vi "Allan variance.vi"(9 "iTime":sgl[](array[numeric])=[1.0, 2.0, 5.0, 10.0, 20.0, 25.0, 50.0, 100.0, 200.0, 250.0, 500.0, 1000.0], 10 "mTime":sgl=1.0, 11 "Data In":sgl[](array[numeric])) -> (3 "Allan Variances":cluster{"iTime":sgl[], sgl[]}(graph))   [LabVIEW 2014, in "Math Utilities.lvlib"]
doc: "This VI produces Allan variance plots of sequential data. The Allan variance plots are used to analyze the stability of the measurements over a period of time. They provide an estimate of the stability due to noise processes and not that of systematic errors or imperfections. \n\nThe source that was used to code these calculations is Werle et al. (1993) - \"The Limits of Signal Averaging in Atmospheric Trace Gas Monitoring by Tunable Diode-Laser Absorption Spectroscopy (TDLAS)\" in Applied Physics B."
uses:
  Math Utilities.lvlib
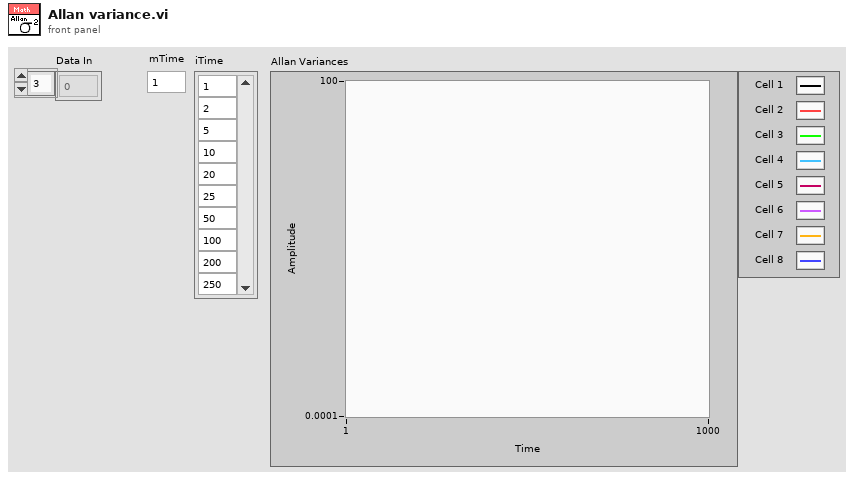
[diagram p1: front panel]
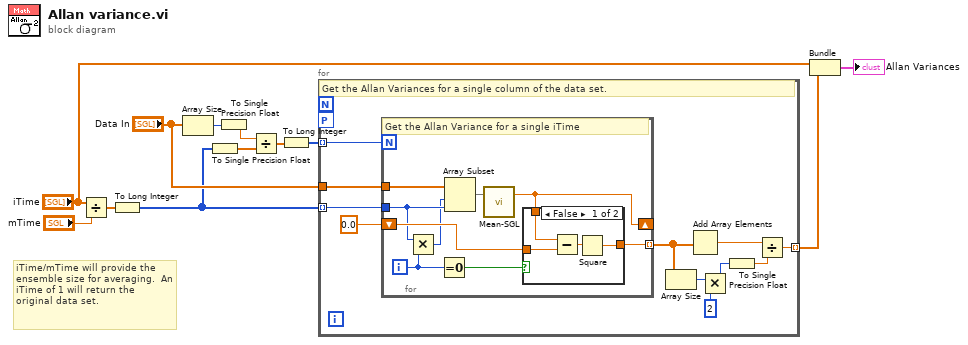
[diagram p0: block diagram]
diagram:
  # "iTime/mTime will provide the ensemble size for averaging.  An iTime of 1 will return the original data set."
  n1 = Divide(x="iTime", y="mTime") -> (x/y=w11:sgl[])
  n2 = To Long Integer(number=w11) -> (32bit integer=w4:i32[])
  n3 = Array Size(array="Data In") -> (size(s)=w6:i32)
  n4 = To Single Precision Float(number=w4) -> (single precision float=w3:sgl[])
  n5 = To Single Precision Float(number=w6) -> (single precision float=w5:sgl)
  n6 = Divide(x=w5, y=w3) -> (x/y=w2:sgl[])
  n7 = To Long Integer(number=w2) -> (32bit integer=w1:i32[])
  n8 = for {
    tunnel: "Data In" -> [w15]
    tunnel: w4 -> [w16] mode=indexing
    tunnel: [w23] -> w8 mode=indexing
    workers-P: _ -> [_]
    tunnel: w1 -> [w14] mode=indexing
    # "Get the Allan Variances for a single column of the data set."
    n9 = for {
      N: w14 -> [_]
      tunnel: w16 -> [w25]
      shift-right: [w29] -> _
      shift-left: sgl 0.0 ("mean") -> [w31]
      tunnel: [w30] -> w21 mode=indexing
      tunnel: w15 -> [w28]
      i -> [w26]
      # "Get the Allan Variance for a single iTime"
      n10 = Multiply(x=w25, y=w26) -> (x*y=w24:i32)
      n11 = Equal To 0?(x=w26) -> (x = 0?=w32:bool)
      n12 = Array Subset(array=w28, index=w24, length=w25) -> (w27:sgl[])
      n13 = call "Mean-SGL.vi"("Data"=w27) -> ("Mean"=w29:sgl)  [unwired: 2 in]
      n14 = case shown="False" w32 {
        tunnel: w31 -> [w36 w37]
        tunnel: w29 -> [w35 _]
        tunnel: [w33 w37] -> w30
        frame False {
          n15 = Subtract(x=w35, y=w36) -> (x-y=w34:sgl)
          n16 = Square(x=w34) -> (x^2=w33:sgl)
        }
        frame True {
        }
      }
    }
    n17 = Array Size(array=w21) -> (size(s)=w20:i32)
    n18 = Add Array Elements(numeric array=w21) -> (sum=w13:sgl)
    n19 = Multiply(x=w20, y=2) -> (x*y=w18:i32)
    n20 = To Single Precision Float(number=w18) -> (single precision float=w17:sgl)
    n21 = Divide(x=w13, y=w17) -> (x/y=w23:sgl)
  }
  n22 = Bundle("iTime"="iTime", w8) -> (→"Allan Variances":cluster{"iTime":sgl[], sgl[]})  [unwired: 1 in]
